vi "Destroy Event.vi"(4 "Error In":errorcluster) -> (0 "Error Out":errorcluster)   [LabVIEW 2014, in "Change Source.lvlib"]
uses:
  Change Source.lvlib
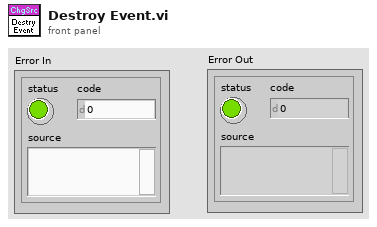
[diagram p1: front panel]
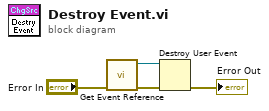
[diagram p0: block diagram]
diagram:
  n1 = call "Get Event Reference.vi"("error in (no error)"="Error In") -> ("error out"=w4:errorcluster, "Event Name"=w3:refnum<user-event>)  [unwired: 5 in]
  n2 = Destroy User Event(user event=w3, error in=w4) -> (error out=→"Error Out":errorcluster)
